vi "Stop.vi"(7 "Emergency Stop? (F)":bool, 8 "error in (no error)":errorcluster, 9 "Wait for Stop Timeout (0 - do not wait)":i32, 11 "API-Reference in":refnum<data-value>) -> (0 "error out":errorcluster, 1 "Timeout":bool, 2 "Final State":refnum<class "Actor.lvclass">)   [LabVIEW 2018, in "Scripting.lvlib" / "Actor.lvclass"]
uses:
  Actor.lvclass
  API-Data.ctl
  Front-Panel State.ctl
  Message-Enqueuer References.ctl
  Stop.ctl
  Launch.ctl
  Did Initialize.ctl
  Did Stop.ctl
  <vilib>/event_ctls.llb/usereventprio.ctl
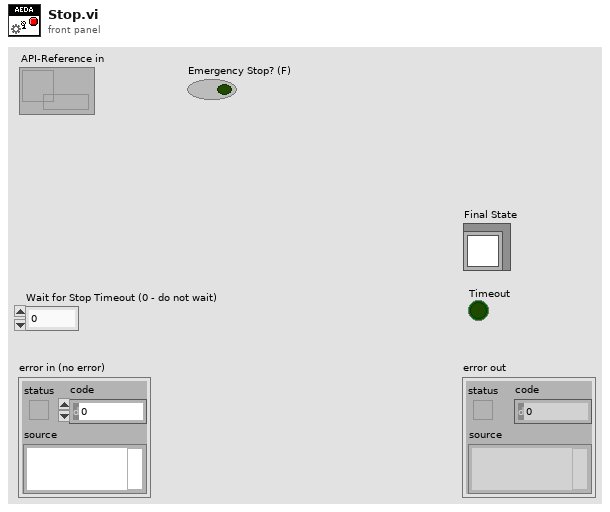
[diagram p1: front panel]
types:
  T1 = typedef "Scripting.lvlib/Actor.lvclass/API-Data.ctl" = cluster{"Launch":refnum<notifier>, "API":T2, "Did Stop Message":refnum<event-registration>, "Did Stop Enqueuer":refnum<user-event>}
  T2 = typedef "Scripting.lvlib/Actor.lvclass/Message-Enqueuer References.ctl" = cluster{"Stop":refnum<user-event>, "Launch":refnum<user-event>, "Did Initialize":refnum<user-event>}
  T3 = typedef "Scripting.lvlib/Actor.lvclass/Stop.ctl" = cluster{"Type":enum16{"Normal", "Emergency"}}
  T4 = typedef "usereventprio.ctl" = enum32{"high priority", "normal priority"}
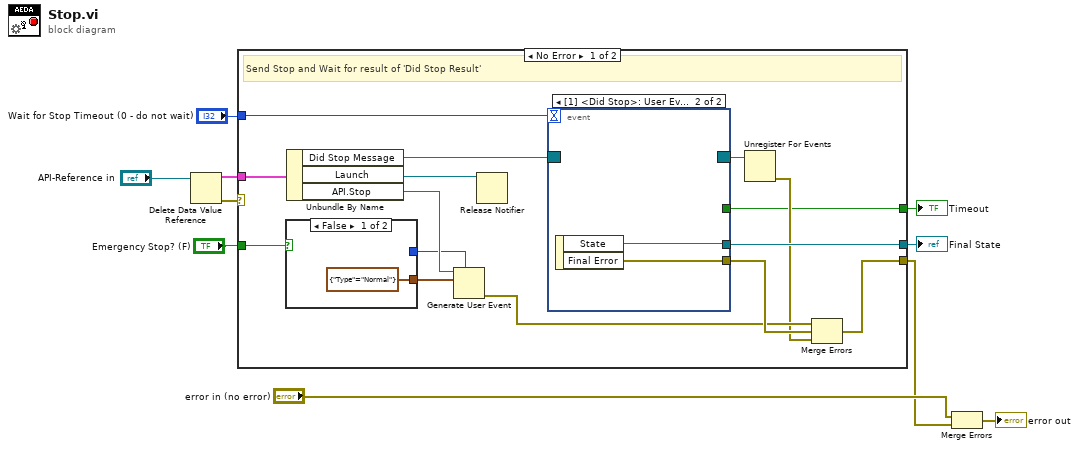
[diagram p0: block diagram]
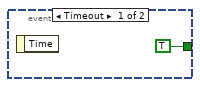
[diagram p2: hidden frame]
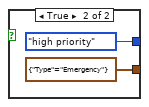
[diagram p3: hidden frame]
diagram:
  n1 = Delete Data Value Reference(data value reference="API-Reference in") -> (data value=w8:T1, error out=w7:errorcluster)  [unwired: 1 in]
  n2 = case shown="No Error" w7 {
    selector: w7 -> [_ w32]
    tunnel: w8 -> [w25 _]
    tunnel: [w14 w32] -> w3
    tunnel: "Emergency Stop? (F)" -> [w24 _]
    tunnel: "Wait for Stop Timeout (0 - do not wait)" -> [w19 _]
    tunnel: [w16 _] -> w5
    tunnel: [w11 _] -> w1
    frame No Error {
      # "Send Stop and Wait for result of 'Did Stop Result'"
      n3 = case shown="False" w24 {
        tunnel: [T3 {"Type"=enum."Normal"} ("Stop") T3 {"Type"=enum."Emergency"} ("Stop")] -> w22
        tunnel: [_ usereventprio."high priority" ("priority (normal)")] -> w21
        frame False {
        }
        frame True {
        }
      }
      n4 = Unbundle By Name(w25) -> ("Did Stop Message"=w18:refnum<event-registration>, "Launch"=w20:refnum<notifier>, "API.Stop"=w23:refnum<user-event>)
      n5 = Generate User Event(priority (normal)=w21, user event=w23, event data cluster=w22) -> (error out=w13:errorcluster)  [unwired: 1 in, 1 out]
      n6 = Release Notifier(notifier=w20) -> ()  [unwired: 2 in, 3 out]
      n7 = event shown="[1] <Did Stop>: User Event" {
        selector: w18 -> [_ _]
        dyn-events: [_ _] -> w17
        timeout: w19 -> [_ _]
        tunnel: [_ w28] -> w16
        tunnel: [_ w27] -> w15
        tunnel: [TRUE _] -> w11
        event Timeout {
          n8 = event-data() -> ()  [unwired: 1 in, 1 out]
        }
        event User Event {
          n9 = event-data() -> ("State"=w28:refnum<class "Actor.lvclass">, "Final Error"=w27:errorcluster)  [unwired: 1 in]
        }
      }
      n10 = Unregister For Events(event registration refnum=w17) -> (error out=w12:errorcluster)  [unwired: 1 in]
      n11 = Merge Errors(w13, w15, w12) -> (w14:errorcluster)
    }
    frame Error {
      # "Stop has already been sent!"
    }
  }
  "Final State" <- w5
  "Timeout" <- w1
  n12 = Merge Errors("error in (no error)", w3) -> (→"error out":errorcluster)
